vi "循环扫描脚本.vi"(1 "4-wire":bool, 2 "扫描":T1 {"测试参数"."反向极限电流(mA)" min=0.0 max=3000.0; "测试参数"."反向电压(V)" min=0.0 max=40.0; "测试参数"."电压改变量(V)" min=0.0 max=40.0 step=5e-06; "测试参数"."正向极限电流(mA)" min=0.0 max=3000.0; "测试参数"."正向电压(V)" min=0.0 max=40.0}) -> (0 "Script":string)   [LabVIEW 2021]
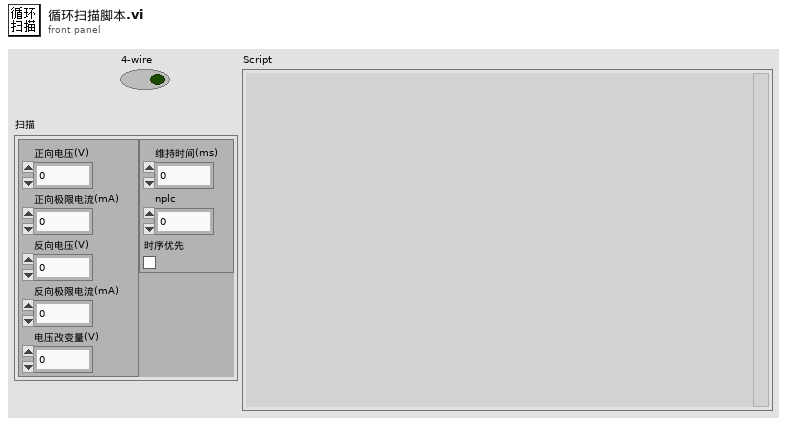
[diagram p1: front panel]
types:
  T1 = typedef "扫描参数.ctl" = cluster{"测试参数":cluster{"正向电压(V)":dbl, "正向极限电流(mA)":dbl, "反向电压(V)":dbl, "反向极限电流(mA)":dbl, "电压改变量(V)":dbl}, "时序参数":cluster{"维持时间(ms)":dbl, "nplc":dbl, "时序优先":bool}}
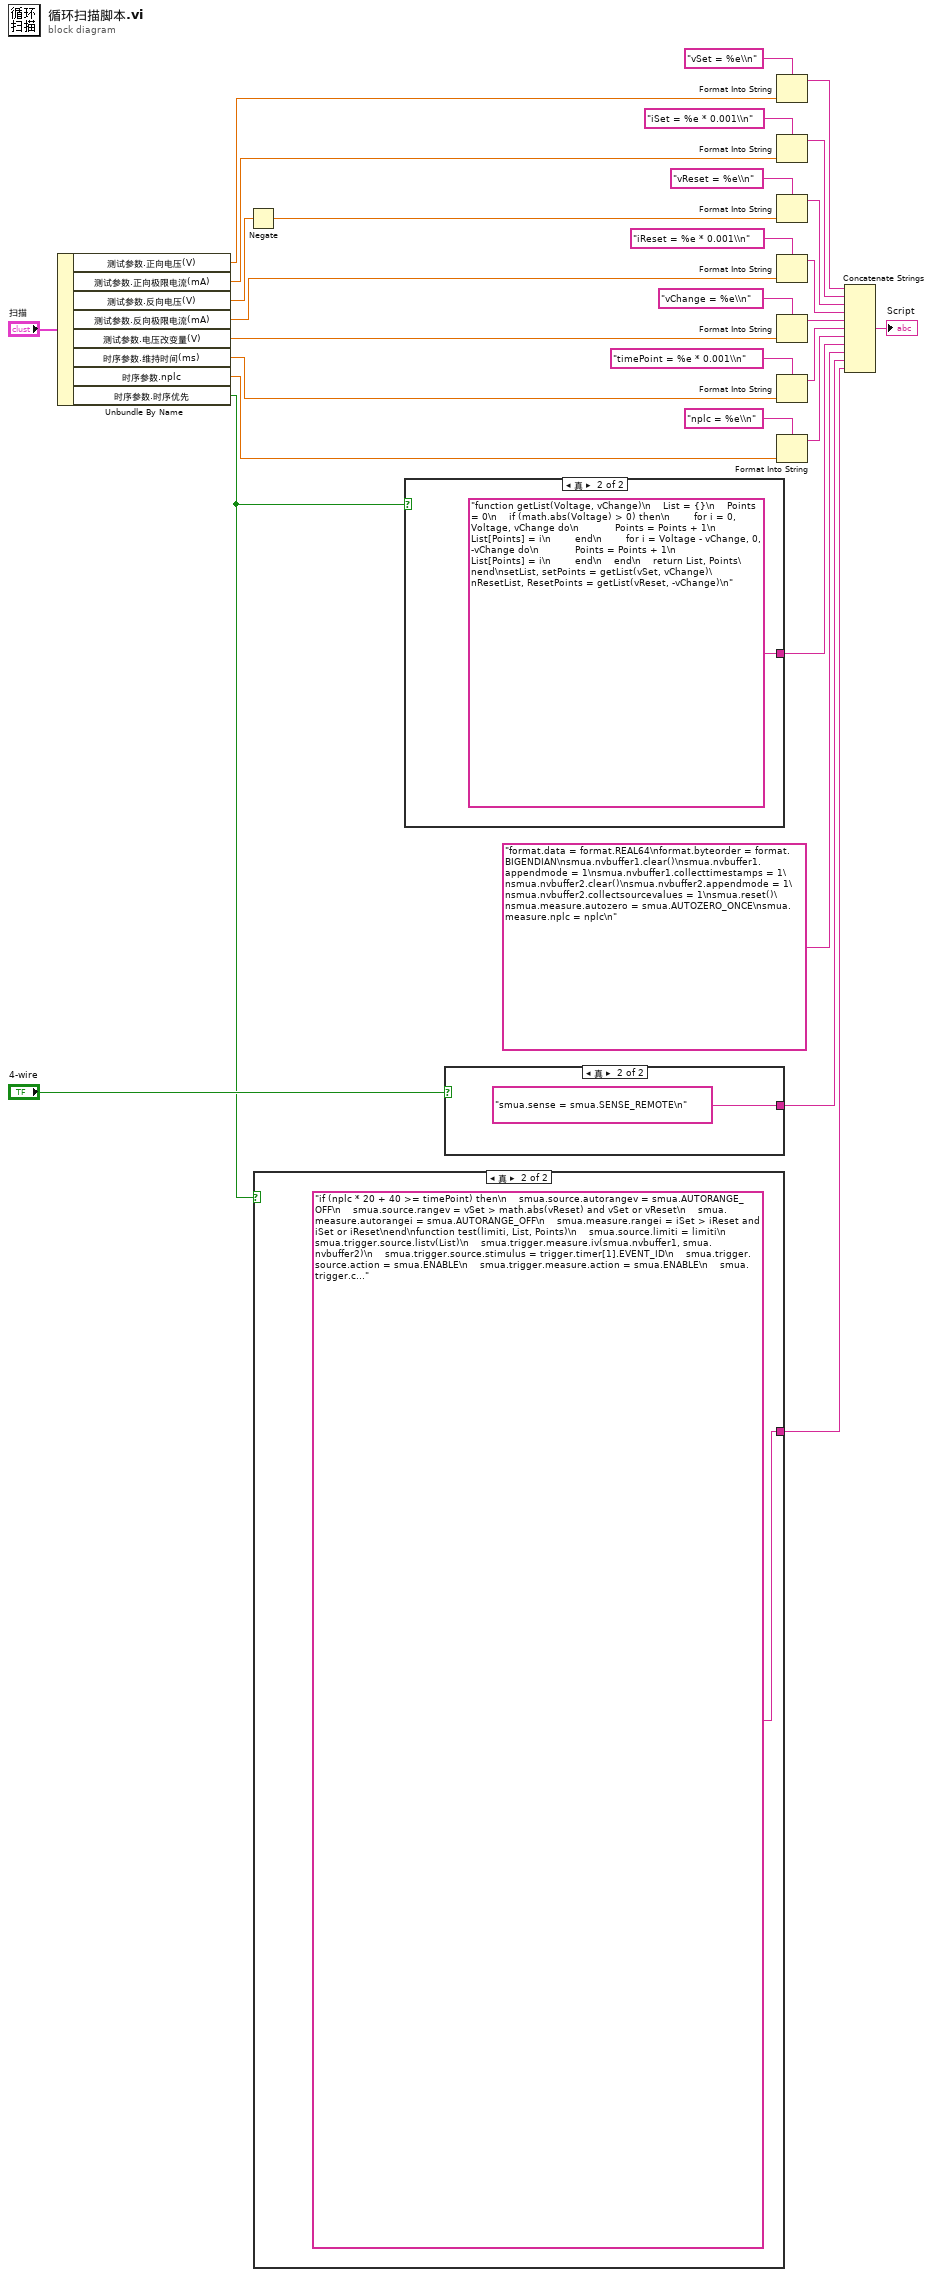
[diagram p0: block diagram]
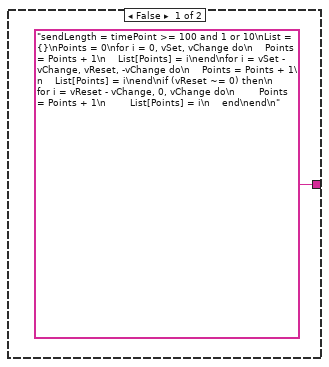
[diagram p2: hidden frame]
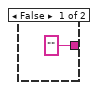
[diagram p3: hidden frame]
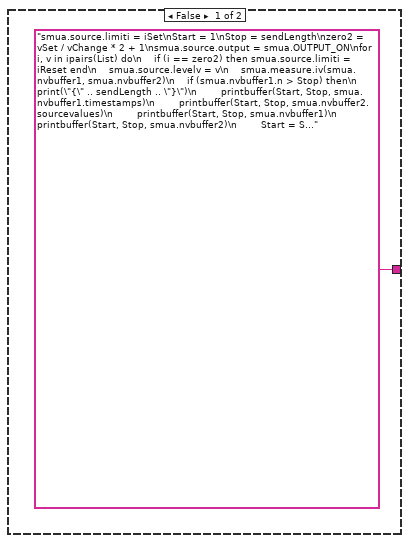
[diagram p4: hidden frame]
diagram:
  n1 = Unbundle By Name("扫描") -> ("测试参数.正向电压(V)"=w7:dbl, "测试参数.正向极限电流(mA)"=w6:dbl, "测试参数.反向电压(V)"=w5:dbl, "测试参数.反向极限电流(mA)"=w4:dbl, "测试参数.电压改变量(V)"=w3:dbl, "时序参数.维持时间(ms)"=w12:dbl, "时序参数.nplc"=w13:dbl, "时序参数.时序优先"=w1:bool)
  n2 = Negate(x=w5) -> (-x=w2:dbl)
  n3 = case shown="真" w1 {
    tunnel: ["smua.source.limiti = iSet\nStart = 1\nStop = sendLength\nzero2 = vSet / vChange * 2 + 1\nsmua.source.output = smua.OUTPUT_ON\nfor i, v in ipairs(List) do\n    if (i == zero2) then smua.source.limiti = iReset end\n    smua.source.levelv = v\n    smua.measure.iv(smua.nvbuffer1, smua.nvbuffer2)\n    if (smua.nvbuffer1.n > Stop) then\n        print(\"{\" .. sendLength .. \"}\")\n        printbuffer(Start, Stop, smua.nvbuffer1.timestamps)\n        printbuffer(Start, Stop, smua.nvbuffer2.sourcevalues)\n        printbuffer(Start, Stop, smua.nvbuffer1)\n        printbuffer(Start, Stop, smua.nvbuffer2)\n        Start = Start + sendLength\n        Stop = Stop + sendLength\n    end\nend\nsmua.source.output = smua.OUTPUT_OFF\nStop = Points\nprint(\"{\" .. Stop - Start + 1 .. \"}\")\nprintbuffer(Start, Stop, smua.nvbuffer1.timestamps)\nprintbuffer(Start, Stop, smua.nvbuffer2.sourcevalues)\nprintbuffer(Start, Stop, smua.nvbuffer1)\nprintbuffer(Start, Stop, smua.nvbuffer2)\nprint(\"{done}\")\nreset()" "if (nplc * 20 + 40 >= timePoint) then\n    smua.source.autorangev = smua.AUTORANGE_OFF\n    smua.source.rangev = vSet > math.abs(vReset) and vSet or vReset\n    smua.measure.autorangei = smua.AUTORANGE_OFF\n    smua.measure.rangei = iSet > iReset and iSet or iReset\nend\nfunction test(limiti, List, Points)\n    smua.source.limiti = limiti\n    smua.trigger.source.listv(List)\n    smua.trigger.measure.iv(smua.nvbuffer1, smua.nvbuffer2)\n    smua.trigger.source.stimulus = trigger.timer[1].EVENT_ID\n    smua.trigger.source.action = smua.ENABLE\n    smua.trigger.measure.action = smua.ENABLE\n    smua.trigger.count = Points\n    smua.trigger.arm.stimulus = trigger.EVENT_ID\n    trigger.timer[1].reset()\n    trigger.timer[1].stimulus = smua.trigger.ARMED_EVENT_ID\n    trigger.timer[1].passthrough = false\n    trigger.timer[1].delay = timePoint\n    trigger.timer[1].count = Points\n    smua.trigger.initiate()\n    smua.trigger.arm.set()\nend\nfunction sendData()\n    repeat\n        if (bit.test(status.operation.instrument.smua.condition, 4) == false) then\n            return\n        elseif (smua.nvbuffer1.n > Stop) then\n            print(\"{\" .. sendLength .. \"}\")\n            printbuffer(Start, Stop, smua.nvbuffer1.timestamps)\n            printbuffer(Start, Stop, smua.nvbuffer2.sourcevalues)\n            printbuffer(Start, Stop, smua.nvbuffer1)\n            printbuffer(Start, Stop, smua.nvbuffer2)\n            Start = Start + sendLength\n            Stop = Stop + sendLength\n        end\n        delay(timePoint)\n    until (false)\nend\nfunction sendLastData()\n    Stop = smua.nvbuffer1.n\n    print(\"{\" .. Stop - Start + 1 .. \"}\")\n    printbuffer(Start, Stop, smua.nvbuffer1.timestamps)\n    printbuffer(Start, Stop, smua.nvbuffer2.sourcevalues)\n    printbuffer(Start, Stop, smua.nvbuffer1)\n    printbuffer(Start, Stop, smua.nvbuffer2)\n    print(\"{done}\")\nend\nStart = 1\nStop = sendLength\nsmua.source.output = smua.OUTPUT_ON\nif (setPoints > 0) then\n    test(iSet, setList, setPoints)\n    sendData()\nend\nif (ResetPoints > 0) then\n    test(iReset, ResetList, ResetPoints)\n    sendData()\nend\nsmua.source.output = smua.OUTPUT_OFF\nsendLastData()\nreset()"] -> w22
    frame False {
    }
    frame True {
    }
  }
  n4 = case shown="真" w1 {
    tunnel: ["sendLength = timePoint >= 100 and 1 or 10\nList = {}\nPoints = 0\nfor i = 0, vSet, vChange do\n    Points = Points + 1\n    List[Points] = i\nend\nfor i = vSet - vChange, vReset, -vChange do\n    Points = Points + 1\n    List[Points] = i\nend\nif (vReset ~= 0) then\n    for i = vReset - vChange, 0, vChange do\n        Points = Points + 1\n        List[Points] = i\n    end\nend\n" "function getList(Voltage, vChange)\n    List = {}\n    Points = 0\n    if (math.abs(Voltage) > 0) then\n        for i = 0, Voltage, vChange do\n            Points = Points + 1\n            List[Points] = i\n        end\n        for i = Voltage - vChange, 0, -vChange do\n            Points = Points + 1\n            List[Points] = i\n        end\n    end\n    return List, Points\nend\nsetList, setPoints = getList(vSet, vChange)\nResetList, ResetPoints = getList(vReset, -vChange)\n"] -> w23
    frame False {
    }
    frame True {
    }
  }
  n5 = case shown="真" "4-wire" {
    tunnel: ["" "smua.sense = smua.SENSE_REMOTE\n"] -> w21
    frame False {
    }
    frame True {
    }
  }
  n6 = Format Into String(format string="vSet = %e\\n" ("格式字符串"), w7) -> (resulting string=w9:string)  [unwired: 2 in, 1 out]
  n7 = Format Into String(format string="iSet = %e * 0.001\\n" ("格式字符串"), w6) -> (resulting string=w8:string)  [unwired: 2 in, 1 out]
  n8 = Format Into String(format string="vReset = %e\\n" ("格式字符串"), w2) -> (resulting string=w27:string)  [unwired: 2 in, 1 out]
  n9 = Format Into String(format string="iReset = %e * 0.001\\n" ("格式字符串"), w4) -> (resulting string=w17:string)  [unwired: 2 in, 1 out]
  n10 = Format Into String(format string="vChange = %e\\n" ("格式字符串"), w3) -> (resulting string=w18:string)  [unwired: 2 in, 1 out]
  n11 = Format Into String(format string="timePoint = %e * 0.001\\n", w12) -> (resulting string=w16:string)  [unwired: 2 in, 1 out]
  n12 = Format Into String(format string="nplc = %e\\n", w13) -> (resulting string=w15:string)  [unwired: 2 in, 1 out]
  n13 = Concatenate Strings(w9, w8, w27, w17, w18, w16, w15, w23, "format.data = format.REAL64\nformat.byteorder = format.BIGENDIAN\nsmua.nvbuffer1.clear()\nsmua.nvbuffer1.appendmode = 1\nsmua.nvbuffer1.collecttimestamps = 1\nsmua.nvbuffer2.clear()\nsmua.nvbuffer2.appendmode = 1\nsmua.nvbuffer2.collectsourcevalues = 1\nsmua.reset()\nsmua.measure.autozero = smua.AUTOZERO_ONCE\nsmua.measure.nplc = nplc\n", w21, w22) -> (→"Script":string)
